vi "APICorreoMandar.vi"(0 "Correo":string, 3 "error in":errorcluster) -> ()   [LabVIEW 2025]
uses:
  <vilib>/LabVIEW Open Source Project/OpenSerializer.Base64/Serializer.Base64.lvclass/Serializer.Base64.ctl
  <vilib>/LabVIEW Open Source Project/OpenSerializer.Base64/Write charset.vi
  <vilib>/LabVIEW Open Source Project/OpenSerializer.Base64/Base64_CharSet.vi
  <vilib>/LabVIEW Open Source Project/OpenSerializer.Base64/Encode.vi
  <vilib>/httpClient/POSTBuffer.vi
  <vilib>/LabVIEW Open Source Project/OpenSerializer.Base64/Serializer.Base64.lvclass
  <vilib>/httpClient/LabVIEWHTTPClient.lvlib
panel:
  out "write_response":string
  out "access_token":string
  out "write_url":string
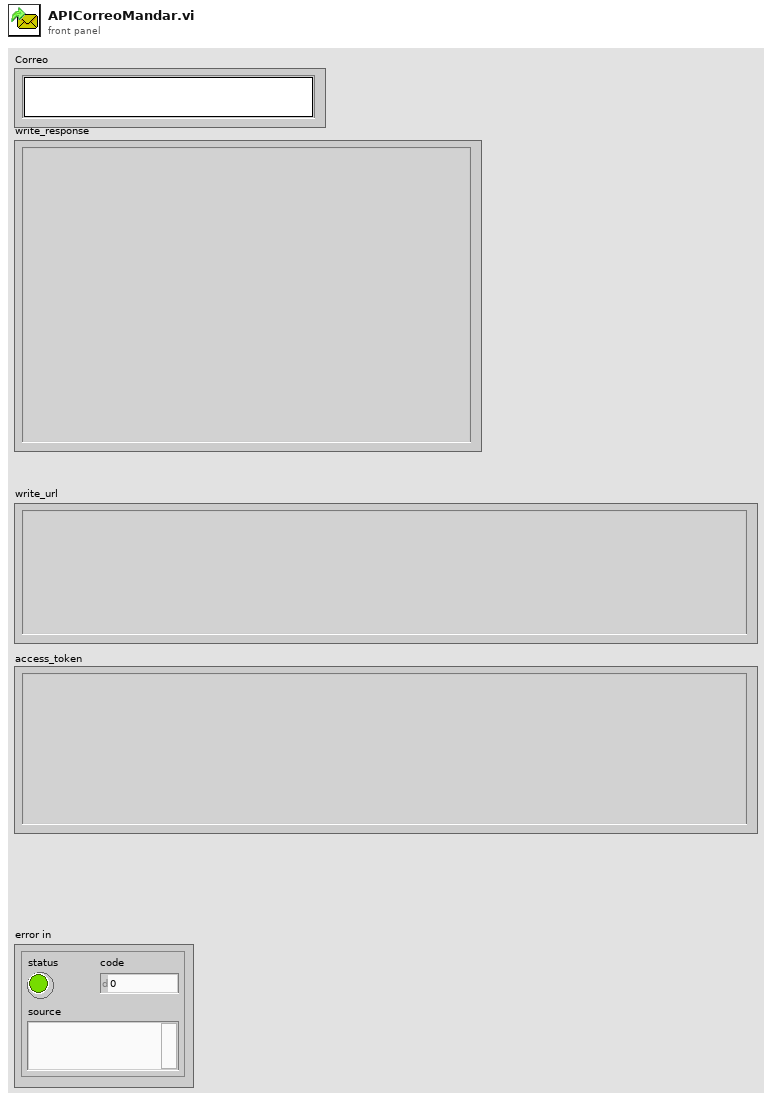
[diagram p1: front panel]
types:
  T1 = typedef "LabVIEWHTTPClient.lvlib/ClientHandle.ctl" = refnum<k1>
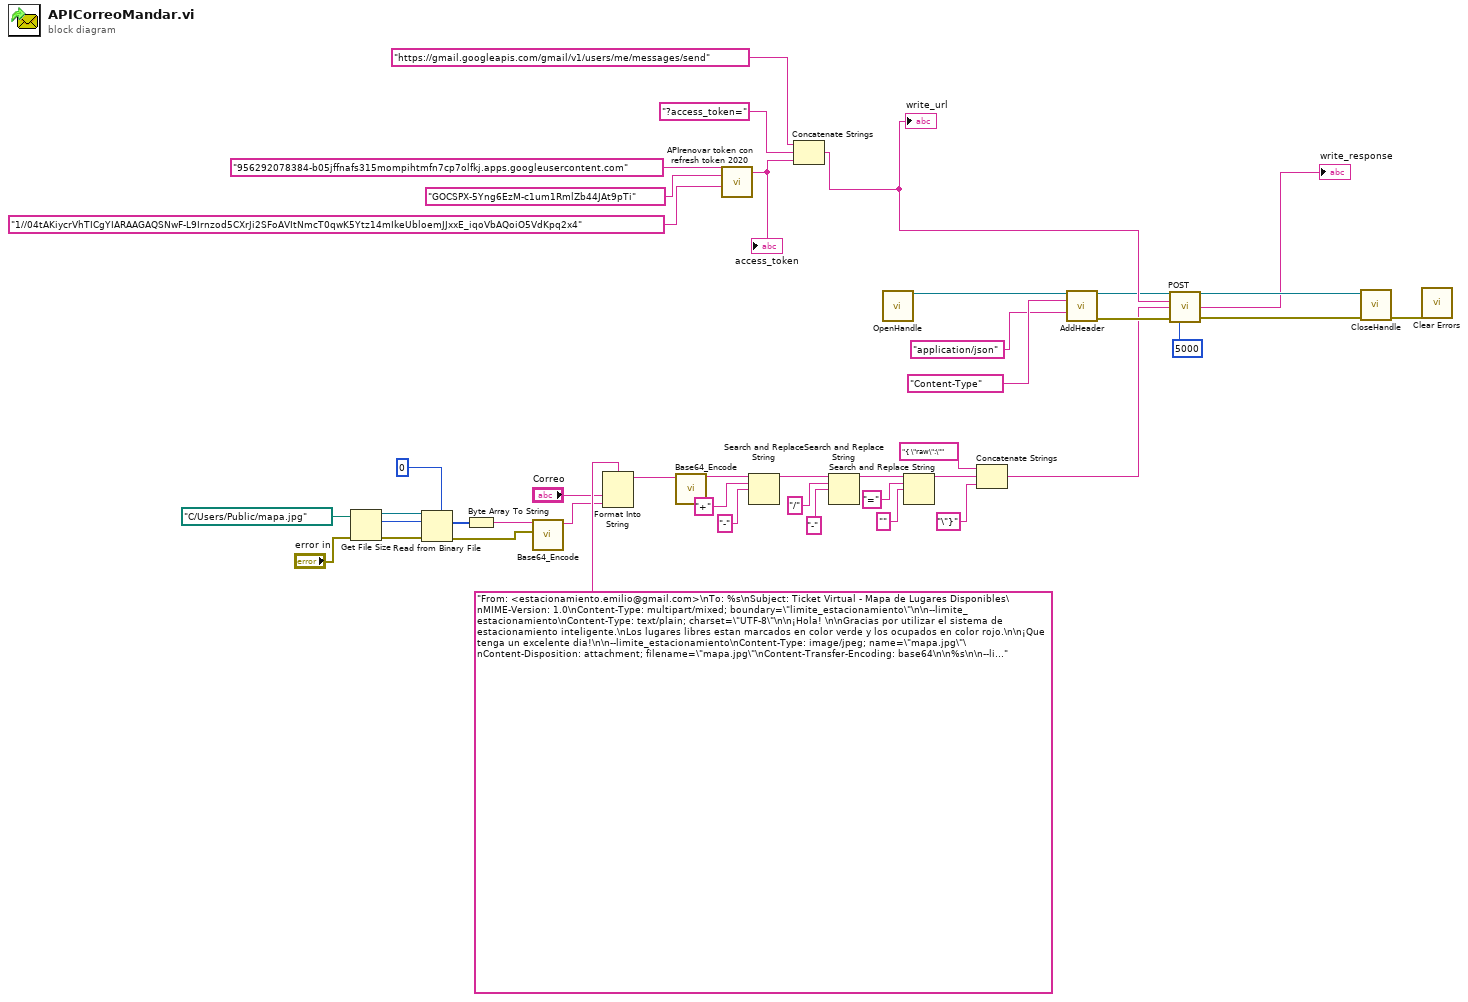
[diagram p0: block diagram]
diagram:
  n1 = Get File Size(file=path "C:/Users/Public/mapa.jpg" ("file (use dialog)"), error in="error in") -> (refnum out=w7:refnum<file>, size (in bytes)=w5:i64, 0:w6:errorcluster)
  n2 = Read from Binary File(5:u8 0, 8:w6, 10:w5, 11:w7) -> (0:w11:errorcluster, 2:w3:u8[])  [unwired: 2 in, 2 out]
  n3 = Byte Array To String(unsigned byte array=w3) -> (string=w10:string)
  n4 = call <vilib>:"Base64_Encode.vi"("error in (no error)"=w11, "String"=w10) -> ("Encoded String"=w13:string)  [unwired: 8 in, 1 out]
  n5 = Format Into String(format string="From: <estacionamiento.emilio@gmail.com>\nTo: %s\nSubject: Ticket Virtual - Mapa de Lugares Disponibles\nMIME-Version: 1.0\nContent-Type: multipart/mixed; boundary=\"limite_estacionamiento\"\n\n--limite_estacionamiento\nContent-Type: text/plain; charset=\"UTF-8\"\n\n¡Hola! \n\nGracias por utilizar el sistema de estacionamiento inteligente.\nLos lugares libres estan marcados en color verde y los ocupados en color rojo.\n\n¡Que tenga un excelente dia!\n\n--limite_estacionamiento\nContent-Type: image/jpeg; name=\"mapa.jpg\"\nContent-Disposition: attachment; filename=\"mapa.jpg\"\nContent-Transfer-Encoding: base64\n\n%s\n\n--limite_estacionamiento--", "Correo", w13) -> (resulting string=w12:string)  [unwired: 2 in, 1 out]
  n6 = call <vilib>:"Base64_Encode.vi"("String"=w12) -> ("Encoded String"=w28:string)  [unwired: 9 in, 1 out]
  n7 = call "APIrenovar token con refresh token 2020.vi"("refresh_token"="1//04tAKiycrVhTICgYIARAAGAQSNwF-L9Irnzod5CXrJi2SFoAVItNmcT0qwK5Ytz14mIkeUbloemJJxxE_iqoVbAQoiO5VdKpq2x4", "client_secret"="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", "client_id"="956292078384-b05jffnafs315mompihtmfn7cp7olfkj.apps.googleusercontent.com") -> ("access_token"=w29:string)  [unwired: 8 in]
  "access_token" <- w29
  n8 = Search and Replace String(input string=w28, search string="+" ("replace string (\"\")"), replace string="-" ("replace string (\"\")")) -> (result string=w27:string)  [unwired: 5 in, 3 out]
  n9 = Concatenate Strings("https://gmail.googleapis.com/gmail/v1/users/me/messages/send", "?access_token=" ("string"), w29) -> (w42:string)
  "write_url" <- w42
  n10 = Search and Replace String(input string=w27, search string="/" ("replace string (\"\")"), replace string="-" ("replace string (\"\")")) -> (result string=w26:string)  [unwired: 5 in, 3 out]
  n11 = call <vilib>:"OpenHandle.vi"() -> ("client handle out"=w32:T1)  [unwired: 14 in, 1 out]
  n12 = Search and Replace String(input string=w26, search string="=" ("replace string (\"\")"), replace string="" ("replace string (\"\")")) -> (result string=w25:string)  [unwired: 5 in, 3 out]
  n13 = Concatenate Strings("{ \"raw\":\"" ("string"), w25, "\"}" ("string")) -> (w16:string)
  n14 = call <vilib>:"AddHeader.vi"("client handle"=w32, "header"="Content-Type", "value"="application/json") -> ("client handle out"=w34:T1, "error out"=w33:errorcluster)  [unwired: 11 in]
  n15 = call-poly <vilib>:"POST.vi"("client handle"=w34, "url"=w42, "buffer"=w16, "error in (no error)"=w33, "timeout (10000)"=5000) -> ("client handle out"=w41:T1, "body"=→"write_response":string, "error out"=w40:errorcluster)  [unwired: 7 in, 1 out]
  n16 = call <vilib>:"CloseHandle.vi"("client handle"=w41, "error in (no error)"=w40) -> ("error out"=w1:errorcluster)  [unwired: 13 in]
  n17 = call <vilib>:"Clear Errors.vi"("error in (no error)"=w1) -> ()  [unwired: 5 in, 2 out]
